vi "補正測試.vi"() -> ()   [LabVIEW 2015]
uses:
  <vilib>/vision/Measure.llb/Edge Options.ctl
  <vilib>/vision/Measure.llb/Edge Polarity.ctl
  <vilib>/vision/Measure.llb/Straight Edge Options.ctl
  <vilib>/vision/Measure.llb/Straight Edge Process.ctl
  <vilib>/vision/driver/NI_Vision_Acquisition_Software.lvlib
  <vilib>/vision/NI_Vision_Development_Module.lvlib
panel:
  in  "Secondary Line Fit Options":T1={"Number of Lines"=1, "Type"=enum."First Edge Rake", "Min. Score"=10.0, "Max. Score"=1000.0, "Orientation"=0.0, "Angle Range"=45.0, "Angle Tolerance"=1.0, "Step Size"=7, "Min. SNR (db)"=0.0, "Min. Points (%)"=25.0, "Hough Iterations"=5} {"Min. Points (%)" min=0.0 max=100.0; "Min. SNR (db)" min=0.0; "Max. Score" min=0.0 max=1024.0; "Min. Score" min=0.0 max=1024.0 step=1.0}
  in  "Primary Line Fit Options":T1={"Number of Lines"=1, "Type"=enum."First Edge Rake", "Min. Score"=10.0, "Max. Score"=1000.0, "Orientation"=0.0, "Angle Range"=45.0, "Angle Tolerance"=1.0, "Step Size"=7, "Min. SNR (db)"=0.0, "Min. Points (%)"=25.0, "Hough Iterations"=5} {"Min. Points (%)" min=0.0 max=100.0; "Min. SNR (db)" min=0.0; "Max. Score" min=0.0 max=1024.0; "Min. Score" min=0.0 max=1024.0 step=1.0}
  in  "Options":T5={"Direction"=0, "Primary Edge Options"={"Edge Polarity"=0, "Kernel Size"=3, "Width"=3, "Minimum Edge Strength"=10.0, "Interpolation Type"=enum."Bilinear Fixed", "Data Processing Method"=enum."Average"}, "Secondary Edge Options"={"Edge Polarity"=0, "Kernel Size"=3, "Width"=3, "Minimum Edge Strength"=10.0, "Interpolation Type"=enum."Bilinear Fixed", "Data Processing Method"=enum."Average"}, "Show Search Area"=FALSE, "Show Search Lines"=FALSE, "Show Edges Found"=FALSE, "Show Result"=TRUE, "Search Area Color"=65280, "Search Lines Color"=255, "Edge Locations Color"=16776960, "Result Color"=16711680, "Overlay Group Name"=""} {"Secondary Edge Options"."Edge Polarity" items=["All Edges", "Rising Edges", "Falling Edges"]; "Secondary Edge Options"."Minimum Edge Strength" format="%.2f"; "Secondary Edge Options"."Width" step=2; "Secondary Edge Options"."Kernel Size" step=2; "Primary Edge Options"."Edge Polarity" items=["All Edges", "Rising Edges", "Falling Edges"]; "Primary Edge Options"."Minimum Edge Strength" format="%.2f"; "Primary Edge Options"."Width" step=2; "Primary Edge Options"."Kernel Size" step=2}
  in  "Mode":u16(ring) items=["Find Reference", "Update CoordSys"]
  in  "ROIsize":cluster{"Width":dbl, "Height":dbl}[](array[cluster])
  in  "Path Array":path[](array[path])
  in  "ROI數量":i32=1
  in  "Don't need to press Ctrl To ZoomIn/ZoomOut":bool
  in  "Cameraindex":i32
  in  "持續更新":bool
  in  "使用固定圖片":bool
  in  "開圖":bool=TRUE
  in  "影像數量":i32=1
  in  "ImageIndex":i32(slide) min=0 scale=0.0..5.0
  in  "重新開圖":bool
  in  "取像":bool
  out "error out":errorcluster
  in  "stop":bool
  out "Image":T6(plugin-control)
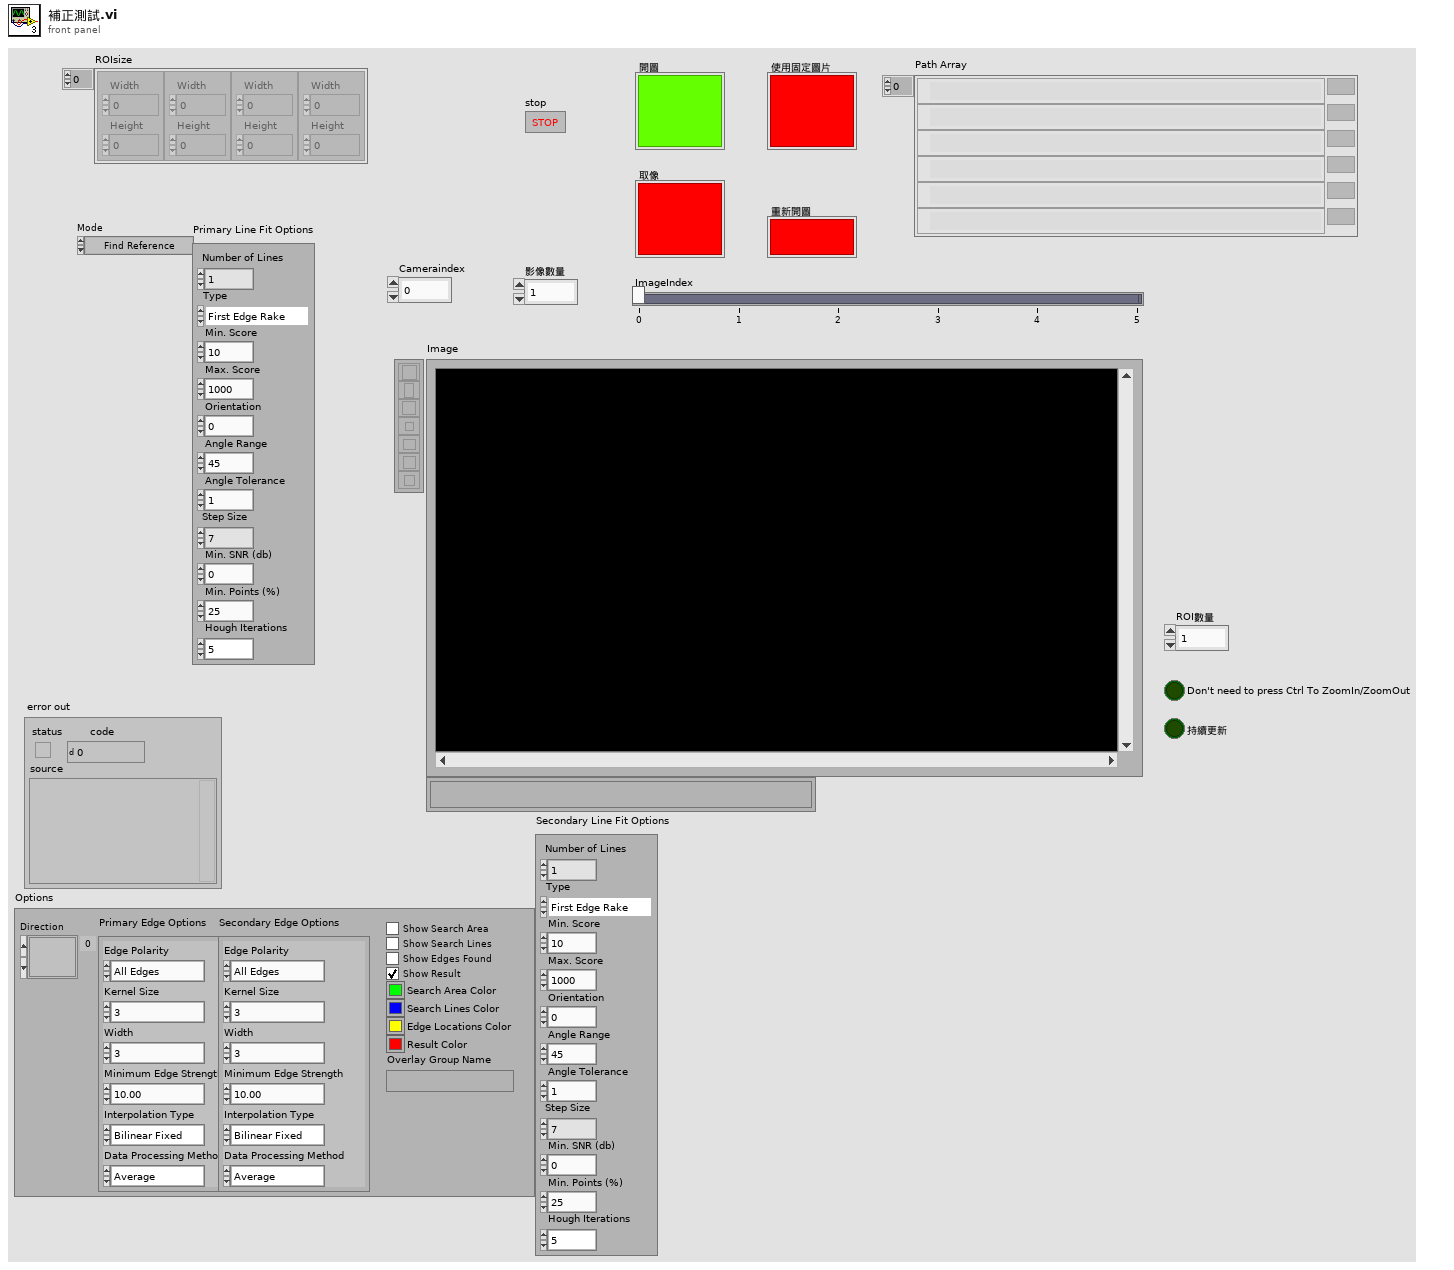
[diagram p1: front panel]
types:
  T1 = typedef "Straight Edge Options.ctl" = cluster{"Number of Lines":i32, "Type":T2, "Min. Score":dbl, "Max. Score":dbl, "Orientation":dbl, "Angle Range":dbl, "Angle Tolerance":dbl, "Step Size":u32, "Min. SNR (db)":dbl, "Min. Points (%)":dbl, "Hough Iterations":i32}
  T2 = typedef "Straight Edge Process.ctl" = enum32{"First Edge Rake", "Best Edge Rake", "Hough Edge Rake", "First Edge Projection", "Best Edge Projection"}
  T3 = typedef "Edge Options.ctl" = cluster{"Edge Polarity":T4, "Kernel Size":u32, "Width":u32, "Minimum Edge Strength":sgl, "Interpolation Type":enum32{"Zero Order", "Bilinear", "Quadratic", "Cubic", "Bilinear Fixed"}, "Data Processing Method":enum32{"Average", "Median"}}
  T4 = typedef "Edge Polarity.ctl" = u32
  T5 = cluster{"Direction":u16, "Primary Edge Options":T3, "Secondary Edge Options":T3, "Show Search Area":bool, "Show Search Lines":bool, "Show Edges Found":bool, "Show Result":bool, "Search Area Color":u32, "Search Lines Color":u32, "Edge Locations Color":u32, "Result Color":u32, "Overlay Group Name":string}
  T6 = typedef "IMAQ Image.ctl" = refnum<image>
  T7 = cluster{"Type":u32, "Version":u32, "Flags":u32, "SerialNumberHigh":u32, "SerialNumberLow":u32, "BusType":u32, "InterfaceName":string, "VendorName":string, "ModelName":string, "CameraFileName":string, "CameraAttributeURL":string}[]
  T8 = typedef "IMAQdx.ctl" = refnum<k21>
  T9 = cluster{"Global Rectangle":i32[], "Contours":cluster{"Contour Type":u32, "ROI Type":u32, "Points":i32[]}[]}
  T10 = cluster{"ROI":cluster{"Global Rectangle":i32[], "Contours":cluster{"Contour Type":u32, "ROI Type":u32, "Points":i32[]}[]}, "ROIsize":cluster{"Width":dbl, "Height":dbl}[], "Options":cluster{"Direction":u16, "Primary Edge Options":T3, "Secondary Edge Options":T3, "Show Search Area":bool, "Show Search Lines":bool, "Show Edges Found":bool, "Show Result":bool, "Search Area Color":u32, "Search Lines Color":u32, "Edge Locations Color":u32, "Result Color":u32, "Overlay Group Name":string}}
  T11 = cluster{"重新開圖":bool, "取像":bool, "Cameraindex":i32, "ImageIndex":i32, cluster{"ROI":cluster{"Global Rectangle":i32[], "Contours":cluster{"Contour Type":u32, "ROI Type":u32, "Points":i32[]}[]}, "ROIsize":cluster{"Width":dbl, "Height":dbl}[], "Options":cluster{"Direction":u16, "Primary Edge Options":T3, "Secondary Edge Options":T3, "Show Search Area":bool, "Show Search Lines":bool, "Show Edges Found":bool, "Show Result":bool, "Search Area Color":u32, "Search Lines Color":u32, "Edge Locations Color":u32, "Result Color":u32, "Overlay Group Name":string}}}
  T12 = typedef "ROI Descriptor" = cluster{"Global Rectangle":i32[], "Contours":cluster{"ID":enum32{"External", "Internal"}, "Type":u32, "Coordinates":i32[]}[]}
  T13 = typedef "Image action.ctl" = enum16{"初始化", "創造記憶體", "寫入圖片", "讀取圖片", "刪除圖片", "等待"}
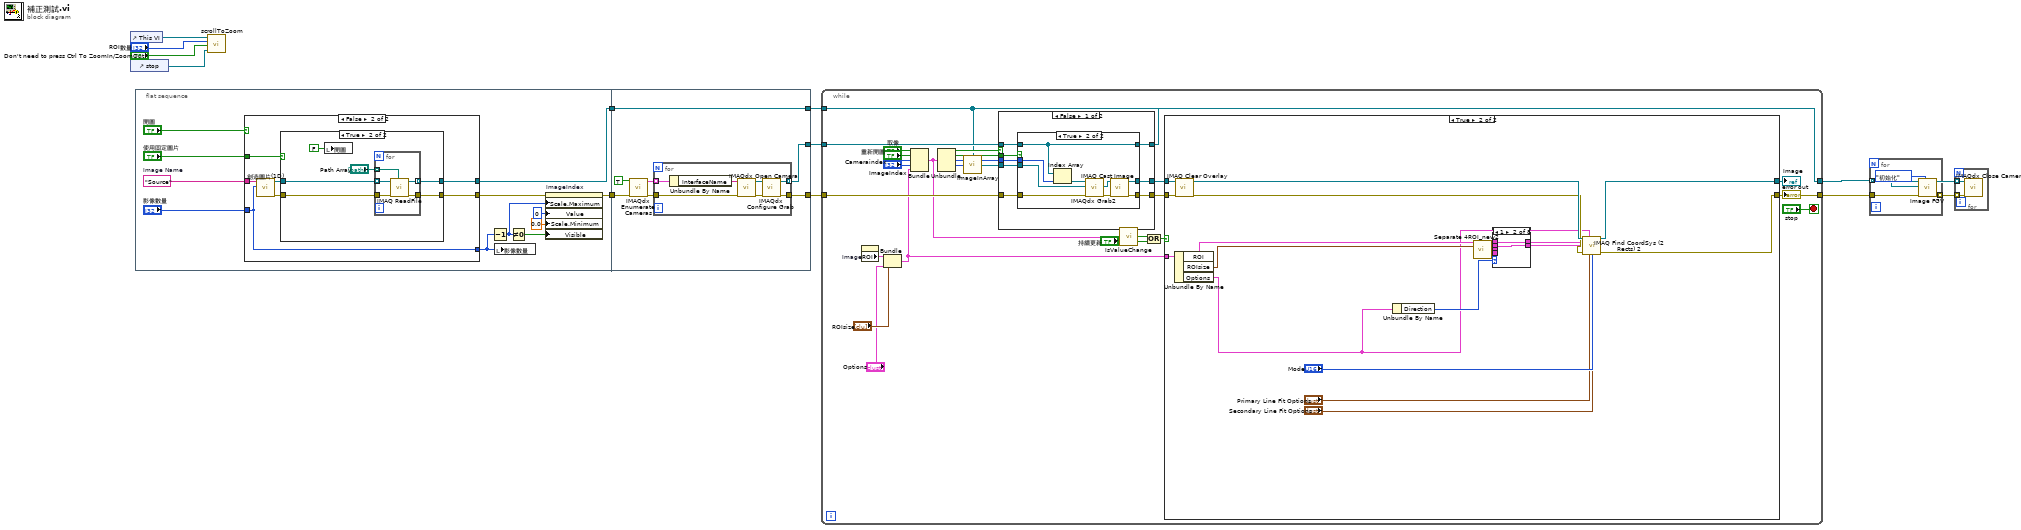
[diagram p0: block diagram]
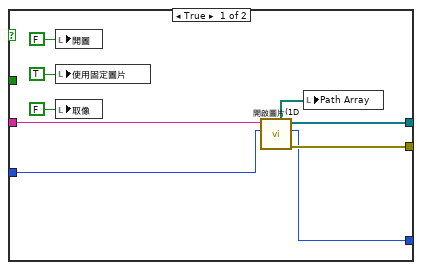
[diagram p2: hidden frame]
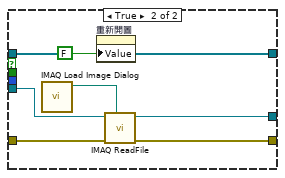
[diagram p5: hidden frame]
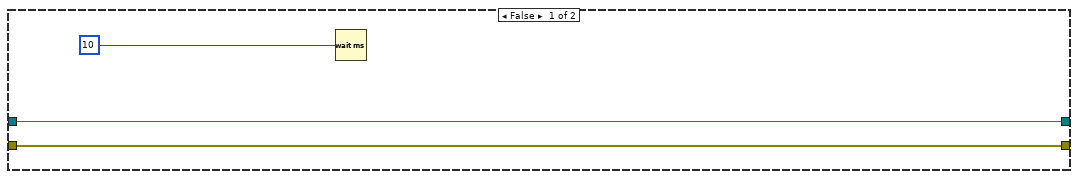
[diagram p6: hidden frame]
diagram:
  n1 = control-ref of="This VI"() -> (w9:refnum<vi>)
  n2 = control-ref of="stop"() -> (w6:refnum<vi>)
  n3 = flat-sequence {
    tunnel: [w18] -> w12
    tunnel: [w25] -> w11
    tunnel: [w55] -> w10
    tunnel: [w61] -> w13
    tunnel: w12 -> [w61]
    tunnel: w11 -> [w58]
    tunnel: [w57] -> w5
    frame #0 {
      w21 = "Source"  # Image Name
      n4 = case shown="False" "開圖" {
        tunnel: w21 -> [w31 w41]
        tunnel: "影像數量" -> [w30 w35]
        tunnel: [w29 w38] -> w19
        tunnel: [w28 w39] -> w18
        tunnel: [w27 w35] -> w14
        tunnel: "使用固定圖片" -> [_ w36]
        frame True {
          n5 = local write "開圖"(FALSE ("取像")) -> ()
          n6 = local write "使用固定圖片"(TRUE ("取像")) -> ()
          n7 = local write "取像"(FALSE ("取像")) -> ()
          n8 = call "開啟圖片(1D.vi"("影像數量"=w30, "Image Name"=w31) -> ("error out"=w29:errorcluster, "ImagePathNumber"=w27:i32, "Image1DArray"=w28:T6[], "ImagePath"=w26:path[])  [unwired: 5 in, 1 out]
          n9 = local write "Path Array"(w26) -> ()
        }
        frame False {
          n10 = call "創造圖片(1D).vi"("影像數量"=w35, "Image Name"=w41) -> ("error out"=w37:errorcluster, "Image1DArray"=w40:T6[])  [unwired: 7 in, 1 out]
          n11 = case shown="True" w36 {
            tunnel: w40 -> [w42 w49]
            tunnel: [w42 w44] -> w39
            tunnel: [w43 w47] -> w38
            tunnel: w37 -> [w43 w46]
            frame False {
            }
            frame True {
              n12 = local write "開圖"(FALSE ("取像")) -> ()
              n13 = for {
                tunnel: w49 -> [w50] mode=indexing
                tunnel: "Path Array" -> [w54] mode=indexing
                tunnel: [w53] -> w44 mode=indexing
                tunnel: w46 -> [w51]
                tunnel: [w52] -> w47
                n14 = call "IMAQ ReadFile"("File Path"=w54, "error in (no error)"=w51, "Image"=w50) -> ("error out"=w52:errorcluster, "Image Out"=w53:T6)  [unwired: 4 in, 3 out]
              }
            }
          }
        }
      }
      n15 = Decrement(x=w14) -> (x-1=w23:i32)
      n16 = local write "影像數量"(w14) -> ()
      n17 = Not Equal To 0?(x=w23) -> (x != 0?=w22:bool)
      n18 = property on="ImageIndex" class="Slide (strict)"(error in=w19, "Scale.Maximum"=w23, "Value"=0 ("Scale.Range:Minimum"), "Scale.Minimum"=0.0 ("Scale.Range:Minimum"), "Visible"=w22) -> (error out=w25:errorcluster)  [unwired: 1 in, 1 out]
    }
    frame #1 {
      n19 = call <vilib>:"IMAQdx Enumerate Cameras.vi"("error in"=w58, "Connected Only? (Yes)"=TRUE ("Connected Only?")) -> ("error out"=w56:errorcluster, "Camera Information Array"=w59:T7)  [unwired: 8 out]
      n20 = for {
        tunnel: w59 -> [w68] mode=indexing
        tunnel: [w64] -> w57 mode=indexing
        tunnel: w56 -> [w66]
        tunnel: [w62] -> w55
        n21 = Unbundle By Name(w68) -> ("InterfaceName"=w67:string)
        n22 = call <vilib>:"IMAQdx Open Camera.vi"("error in"=w66, "Session In"=w67) -> ("error out"=w63:errorcluster, "Session Out"=w65:T8)  [unwired: 1 in, 7 out]
        n23 = call <vilib>:"IMAQdx Configure Grab.vi"("error in"=w63, "Session In"=w65) -> ("error out"=w62:errorcluster, "Session Out"=w64:T8)  [unwired: 8 out]
      }
    }
  }
  n24 = call "scrollToZoom.vi"("stop"=w6, "Don't need to press Ctrl To ZoomIn/ZoomOut"="Don't need to press Ctrl To ZoomIn/ZoomOut", "ROI數量"="ROI數量", "VI in"=w9) -> ()  [unwired: 8 in]
  n25 = while {
    tunnel: w13 -> [w73]
    tunnel: w10 -> [w90]
    tunnel: w5 -> [w87]
    tunnel: [w79] -> w3
    tunnel: [w73] -> w2
    tunnel: [w78] -> w1
    stop <- "stop" stop-if-true
    n26 = property on="Image" class="ImageControl"() -> ("ROI"=w76:T9)  [unwired: 2 in, 2 out]
    n27 = Bundle("ROI"=w76, "ROIsize"="ROIsize", "Options"="Options") -> (w75:T10)  [unwired: 1 in]
    n28 = Bundle("重新開圖"="重新開圖", "取像"="取像", "Cameraindex"="Cameraindex", "ImageIndex"="ImageIndex", w75) -> (w74:T11)  [unwired: 1 in]
    n29 = Unbundle(w74) -> ("重新開圖"=w82:bool, "取像"=w81:bool, "Cameraindex"=w80:i32, "ImageIndex"=w71:i32)  [unwired: 1 out]
    n30 = call "ImageInArray.vi"("index"=w71, "Array"=w73) -> ("Image"=w72:T6)
    n31 = case shown="False" w82 {
      tunnel: [w98 w121] -> w89
      tunnel: w90 -> [w102 w117]
      tunnel: [w99 w118] -> w88
      tunnel: w81 -> [w101 _]
      tunnel: [w100 w116] -> w78
      tunnel: w87 -> [w97 w116]
      tunnel: w80 -> [w96 _]
      tunnel: w72 -> [w95 w115]
      frame False {
        n32 = case shown="True" w101 {
          tunnel: [w104 w109] -> w100
          tunnel: [w103 w114] -> w98
          tunnel: w102 -> [w105 w107]
          tunnel: [w105 w110] -> w99
          tunnel: w97 -> [w104 w109]
          tunnel: w96 -> [_ w108]
          tunnel: w95 -> [w103 w106]
          frame False {
          }
          frame True {
            n33 = Index Array(array=w109, index=w108) -> (element=w111:T8)
            n34 = call <vilib>:"IMAQdx Grab2.vi"("error in"=w107, "Image In"=w106, "Session In"=w111) -> ("error out"=w112:errorcluster, "Image Out"=w113:T6)  [unwired: 5 in, 2 out]
            n35 = call "IMAQ Cast Image"("error in (no error)"=w112, "Image Src"=w113) -> ("error out"=w110:errorcluster, "Image Dst Out"=w114:T6)  [unwired: 8 in]
          }
        }
      }
      frame True {
        n36 = call "IMAQ Load Image Dialog"() -> ("Path"=w119:path)  [unwired: 9 in, 2 out]
        n37 = property on="重新開圖" class="Bool (strict)"("Value"=FALSE ("重新開圖")) -> ()  [unwired: 2 in, 2 out]
        n38 = call "IMAQ ReadFile"("File Path"=w119, "error in (no error)"=w117, "Image"=w115) -> ("error out"=w118:errorcluster, "Image Out"=w121:T6)  [unwired: 4 in, 3 out]
      }
    }
    n39 = call "IsValueChange.vi"("Variant"=w74) -> ("result"=w77:bool)
    n40 = Or(x=w77, y="持續更新") -> (x .or. y?=w91:bool)
    n41 = case shown="True" w91 {
      tunnel: [w123 w134] -> w93
      tunnel: w89 -> [w123 w144]
      tunnel: w88 -> [w122 w143]
      tunnel: [w122 w133] -> w79
      tunnel: w75 -> [_ w142]
      frame False {
        n42 = Wait (ms)(milliseconds to wait=u32 10) -> ()  [unwired: 1 out]
      }
      frame True {
        n43 = Unbundle By Name(w142) -> ("ROI"=w141:T9, "ROIsize"=w140:cluster{"Width":dbl, "Height":dbl}[], "Options"=w125:T5)
        n44 = call "IMAQ Clear Overlay"("error in (no error)"=w143, "Image"=w144) -> ("error out"=w137:errorcluster, "Image Out"=w139:T6)  [unwired: 8 in]
        n45 = Unbundle By Name(w125) -> ("Direction"=w132:u16)
        n46 = call "Separate 4ROI_new2.vi"("ROI Descriptor"=w141, "ROIsize"=w140) -> ("Left ROI"=w131:T12, "Top ROI"=w130:T12, "Right ROI"=w129:T12, "Bottom ROI"=w128:T12)  [unwired: 9 in, 1 out]
        n47 = case shown="1" w132 {
          tunnel: w131 -> [w146 w148 w149 _ _ _ _ w159]
          tunnel: w130 -> [_ w147 w150 w152 w153 _ _ _]
          tunnel: w129 -> [_ _ _ w151 w154 w156 w157 _]
          tunnel: w128 -> [w145 _ _ _ _ w155 w158 w160]
          tunnel: [w146 w148 w150 w152 w154 w156 w158 w160] -> w127
          tunnel: [w145 w147 w149 w151 w153 w155 w157 w159] -> w126
          frame 0, Default {
          }
          frame 1 {
            # "Second"
          }
          frame 2 {
          }
          frame 3 {
          }
          frame 4 {
          }
          frame 5 {
          }
          frame 6 {
          }
          frame 7 {
          }
        }
        n48 = call "IMAQ Find CoordSys (2 Rects) 2"("Image"=w139, "Options"=w125, "Mode"="Mode", "Primary ROI Descriptor"=w127, "Secondary ROI Descriptor"=w126, "error in (no error)"=w137, "Primary Line Fit Options"="Primary Line Fit Options", "Secondary Line Fit Options"="Secondary Line Fit Options") -> ("Image Out"=w134:T6, "error out"=w133:errorcluster)  [unwired: 3 in, 3 out]
      }
    }
    "Image" <- w93
    "error out" <- w79
  }
  n49 = for {
    tunnel: w2 -> [w164] mode=indexing
    tunnel: [w162] -> w4 mode=indexing
    tunnel: w3 -> [w161]
    n50 = call "Image FGV.vi"("Image action"=Image_action."初始化", "error in (no error)"=w161, "Image In"=w164) -> ("error out"=w162:errorcluster)  [unwired: 7 in, 1 out]
  }
  n51 = for {
    tunnel: w1 -> [w166] mode=indexing
    tunnel: w4 -> [w165] mode=indexing
    n52 = call <vilib>:"IMAQdx Close Camera.vi"("error in"=w165, "Session In"=w166) -> ()  [unwired: 9 in, 1 out]
  }
